vi "LED.vi"() -> ()   [LabVIEW 2024]
panel:
  out "return count":u32
  out "LED":bool
  in  "stop":bool
  in  "เปิด/ปิด":bool
  in  "PORT":refnum<visa-resource-name>
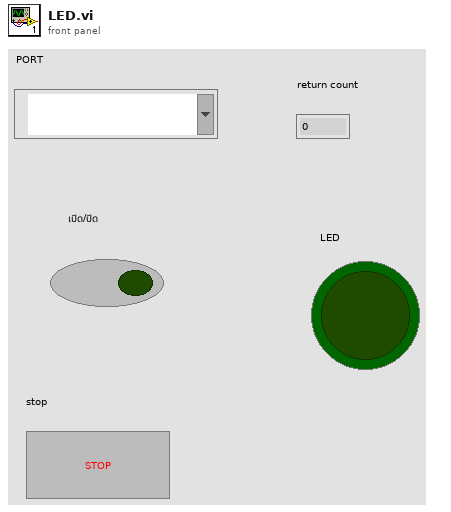
[diagram p1: front panel]
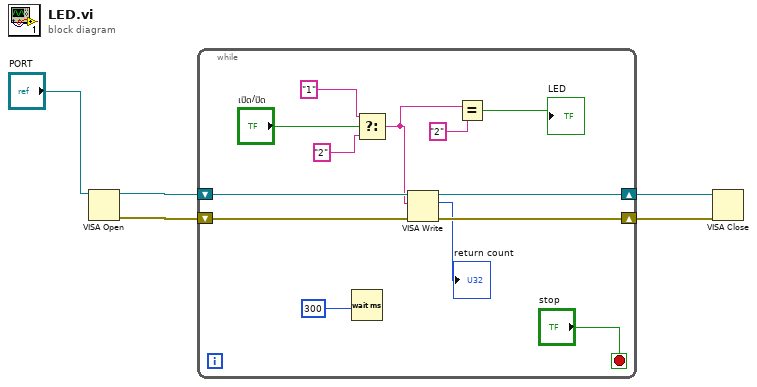
[diagram p0: block diagram]
diagram:
  n1 = VISA Open(VISA resource name="PORT") -> (VISA resource name=w5:refnum<visa-resource-name>, error out=w3:errorcluster)  [unwired: 4 in]
  n2 = while {
    shift-right: [w17] -> w4
    shift-left: w5 -> [w18]
    shift-right: [w15] -> w2
    shift-left: w3 -> [w16]
    stop <- "stop" stop-if-true
    n3 = Wait (ms)(milliseconds to wait=u32 300 ("millisecond timer value")) -> ()  [unwired: 1 out]
    n4 = Select(t="1", s="เปิด/ปิด", f="2") -> (s? t:f=w9:string)
    n5 = VISA Write(VISA resource name=w18, write buffer=w9, error in (no error)=w16) -> (VISA resource name out=w17:refnum<visa-resource-name>, return count=→"return count":u32, error out=w15:errorcluster)
    n6 = Equal?(x=w9, y="2") -> (x = y?=→"LED":bool)
  }
  n7 = VISA Close(VISA resource name=w4, error in (no error)=w2) -> ()  [unwired: 1 out]
